vi "Setup subWorkers.vi"(8 "error in":errorcluster, 11 "Manager Worker in":refnum<class "Manager Worker.lvclass">) -> (0 "error out":errorcluster, 3 "Manager Worker out":refnum<class "Manager Worker.lvclass">)   [LabVIEW 2018, in "Manager Worker.lvclass"]
doc: "<b>Note: Do not change the code in this VI!</b>\nThis VI performs a setup of all the statically-linked subWorkers that belong to the Worker that calls this VI. This VI is created automatically by the 'Create/Add Worker' tool and must be called <b>before</b> any statically linked subWorkers are called."
uses:
  Manager Worker.lvclass
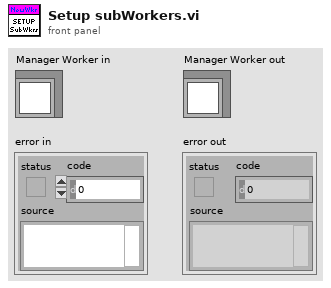
[diagram p1: front panel]
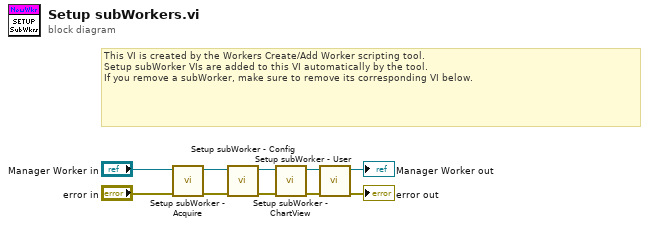
[diagram p0: block diagram]
diagram:
  # "This VI is created by the Workers Create/Add Worker scripting tool.\nSetup subWorker VIs are added to this VI automatically by the tool.\nIf you remove a subWorker, make sure to remove its corresponding VI below."
  n1 = call "Setup subWorker - Acquire.vi"("error in"="error in", "Manager Worker in"="Manager Worker in") -> ("error out"=w9:errorcluster, "Manager Worker out"=w6:refnum<class "Manager Worker.lvclass">)  [unwired: 8 in]
  n2 = call "Setup subWorker - Config.vi"("error in"=w9, "Manager Worker in"=w6) -> ("error out"=w7:errorcluster, "Manager Worker out"=w4:refnum<class "Manager Worker.lvclass">)  [unwired: 8 in]
  n3 = call "Setup subWorker - ChartView.vi"("error in"=w7, "Manager Worker in"=w4) -> ("error out"=w5:errorcluster, "Manager Worker out"=w2:refnum<class "Manager Worker.lvclass">)  [unwired: 8 in]
  n4 = call "Setup subWorker - User.vi"("error in"=w5, "Manager Worker in"=w2) -> ("error out"=→"error out":errorcluster, "Manager Worker out"=→"Manager Worker out":refnum<class "Manager Worker.lvclass">)  [unwired: 8 in]
